vi "overlayCrossAndProfile.vi"(8 "error in (no error)":errorcluster, 10 "Last Mouse P":cluster{"X":i32, "Y":i32}, 11 "ImageStreamViewer in":refnum<class "ImageStreamViewer.lvclass">) -> (0 "error out":errorcluster, 3 "ImageStreamViewer out":refnum<class "ImageStreamViewer.lvclass">)   [LabVIEW 2011, in "Views.lvlib" / "Camera.lvlib" / "ImageStreamViewer.lvclass"]
uses:
  ImageStreamViewer.lvclass
  ImageStreamViewer.lvclass/ImageStreamViewer.ctl
  <vilib>/vision/NI_Vision_Development_Module.lvlib
panel:
  # "At these coordinates overlay two lines, horizontal and\nvertical. And from the image get the image profile along\nthese lines. Display them on the front panel"
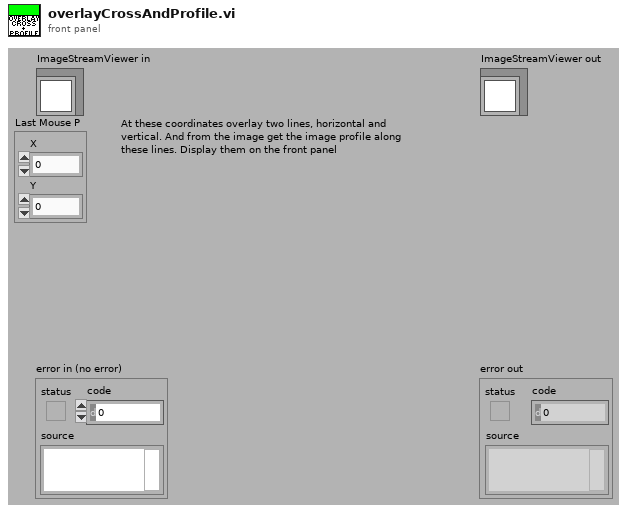
[diagram p1: front panel]
types:
  T1 = typedef "IMAQ Image.ctl" = refnum<image>
  T2 = cluster{"Left":i32, "Top":i32, "Right":i32, "Bottom":i32}
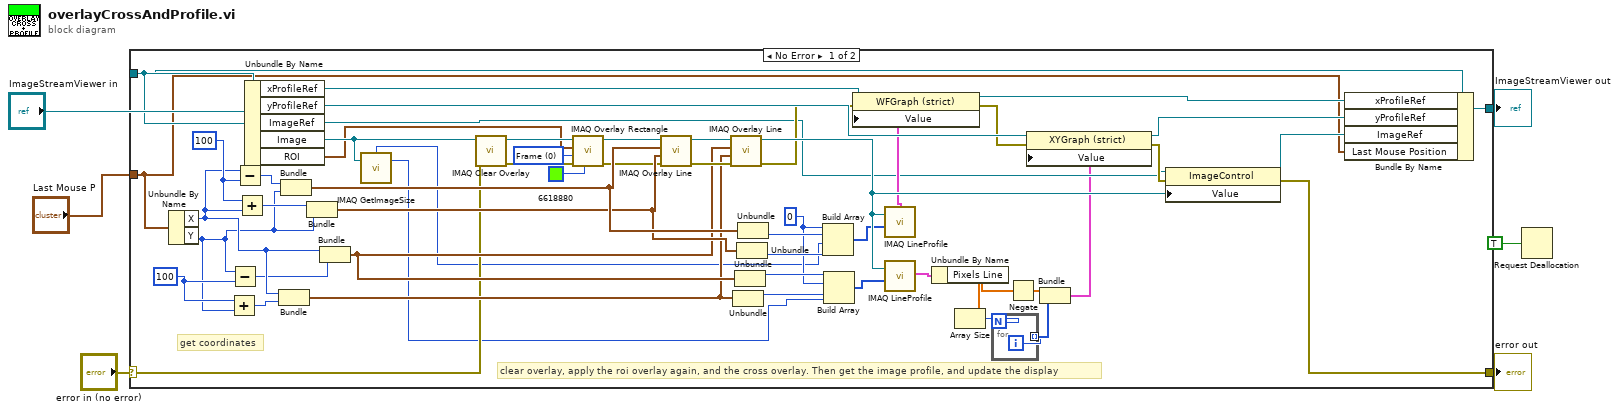
[diagram p0: block diagram]
diagram:
  n1 = case shown="No Error" "error in (no error)" {
    selector: "error in (no error)" -> [w27 w62]
    tunnel: [w29 w62] -> w5
    tunnel: [w56 w61] -> w3
    tunnel: "ImageStreamViewer in" -> [w57 w61]
    tunnel: "Last Mouse P" -> [w17 _]
    frame No Error {
      w8 = u32 0 items=["Frame", "Fill", "Highlight"] ("Drawing Mode (Frame)")
      w25 = 0
      w58 = 100 ("x")
      w59 = 100 ("x")
      # "clear overlay, apply the roi overlay again, and the cross overlay. Then get the image profile, and update the display"
      # "get coordinates"
      n2 = Unbundle By Name(w17) -> ("X"=w51:i32, "Y"=w28:i32)
      n3 = Add(x=w58, y=w28) -> (x+y=w55:i32)
      n4 = Subtract(x=w28, y=w58) -> (x-y=w47:i32)
      n5 = Subtract(x=w51, y=w59) -> (x-y=w48:i32)
      n6 = Add(x=w59, y=w51) -> (x+y=w50:i32)
      n7 = Unbundle By Name(w57) -> ("xProfileRef"=w37:refnum<vi>, "yProfileRef"=w35:refnum<vi>, "ImageRef"=w24:refnum<vi>, "Image"=w10:T1, "ROI"=w9:T2)
      n8 = Bundle("X"=w51, w55) -> (w39:cluster{"X":i32, i32})  [unwired: 1 in]
      n9 = Bundle(w48, "Y"=w28) -> (w46:cluster{i32, "Y":i32})  [unwired: 1 in]
      n10 = Bundle(w50, "Y"=w28) -> (w45:cluster{i32, "Y":i32})  [unwired: 1 in]
      n11 = Bundle("X"=w51, w47) -> (w40:cluster{"X":i32, i32})  [unwired: 1 in]
      n12 = call "IMAQ GetImageSize"("Image"=w10) -> ("Y Resolution"=w16:i32, "X Resolution"=w15:i32)  [unwired: 3 in, 1 out]
      n13 = call "IMAQ Clear Overlay"("error in (no error)"=w27, "Image"=w10) -> ("error out"=w14:errorcluster, "Image Out"=w13:T1)  [unwired: 8 in]
      n14 = call "IMAQ Overlay Rectangle"("Color"=u32 6618880, "error in (no error)"=w14, "Drawing Mode (Frame)"=w8, "Rectangle"=w9, "Image"=w13) -> ("error out"=w11:errorcluster, "Image Out"=w12:T1)  [unwired: 5 in]
      n15 = call "IMAQ Overlay Line"("error in (no error)"=w11, "End Point"=w45, "Start Point"=w46, "Image"=w12) -> ("error out"=w52:errorcluster, "Image Out"=w53:T1)  [unwired: 6 in]
      n16 = call "IMAQ Overlay Line"("error in (no error)"=w52, "End Point"=w39, "Start Point"=w40, "Image"=w53) -> ("error out"=w31:errorcluster, "Image Out"=w49:T1)  [unwired: 6 in]
      n17 = Unbundle(w39) -> ("X"=w41:i32)  [unwired: 1 out]
      n18 = Unbundle(w40) -> ("X"=w42:i32)  [unwired: 1 out]
      n19 = Unbundle(w45) -> ("Y"=w44:i32)  [unwired: 1 out]
      n20 = Unbundle(w46) -> ("Y"=w26:i32)  [unwired: 1 out]
      n21 = Build Array(w25, w26, w15, w44) -> (w43:i32[])
      n22 = Build Array(w42, w25, w41, w16) -> (w38:i32[])
      n23 = call "IMAQ LineProfile"("Line Coordinates"=w43, "Image"=w49) -> ("Line Graph"=w34:cluster{"x0":sgl, "dx":sgl, "Pixels Line":sgl[]})  [unwired: 3 in, 3 out]
      n24 = property class="WFGraph (strict)"(reference=w37, error in=w31, "Value"=w34) -> (reference out=w33:refnum<vi>, error out=w30:errorcluster)
      n25 = call "IMAQ LineProfile"("Line Coordinates"=w38, "Image"=w49) -> ("Line Graph"=w19:cluster{"x0":sgl, "dx":sgl, "Pixels Line":sgl[]})  [unwired: 3 in, 3 out]
      n26 = Unbundle By Name(w19) -> ("Pixels Line"=w20:sgl[])
      n27 = Array Size(array=w20) -> (size(s)=w22:i32)
      n28 = for {
        N: w22 -> [_]
        tunnel: [w60] -> w21 mode=indexing
        i -> [w60]
      }
      n29 = Negate(x=w20) -> (-x=w23:sgl[])
      n30 = Bundle(w23, w21) -> (w18:cluster{sgl[], i32[]})  [unwired: 1 in]
      n31 = property class="XYGraph (strict)"(reference=w35, error in=w30, "Value"=w18) -> (reference out=w32:refnum<vi>, error out=w36:errorcluster)
      n32 = property class="ImageControl"(reference=w24, error in=w36, "Value"=w49) -> (reference out=w54:refnum<vi>, error out=w29:errorcluster)
      n33 = Bundle By Name(cluster=w57, "xProfileRef"=w33, "yProfileRef"=w32, "ImageRef"=w54, "Last Mouse Position"=w17) -> (w56:refnum<class "ImageStreamViewer.lvclass">)
    }
    frame Error {
    }
  }
  "error out" <- w5
  "ImageStreamViewer out" <- w3
  n34 = Request Deallocation(TRUE ("flag")) -> ()
